vi "Test2.vi"(6 "Value":sgl=6.6666, 8 "Path":string=":NUMX", 9 "Mode":string="EDIT", 10 "Shot":i32=-1, 11 "Name":string="my_tree") -> (3 "Float out":sgl)   [LabVIEW 2010]
uses:
  <vilib>/MDSplus/Classes/Tree_Class/Tree.lvclass
  <vilib>/MDSplus/Classes/Data_Class/Scalar_Class/Float32_Class/Float32.lvclass
  <vilib>/MDSplus/Classes/Data_Class/Data.lvclass
  <vilib>/MDSplus/Classes/Data_Class/TreeNode_Class/TreeNode.lvclass
panel:
  out "error out":errorcluster
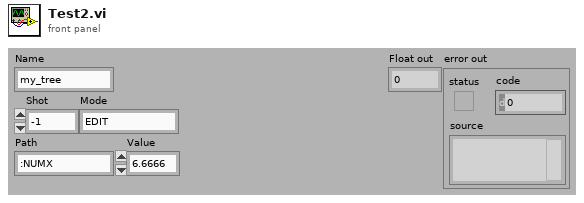
[diagram p1: front panel]
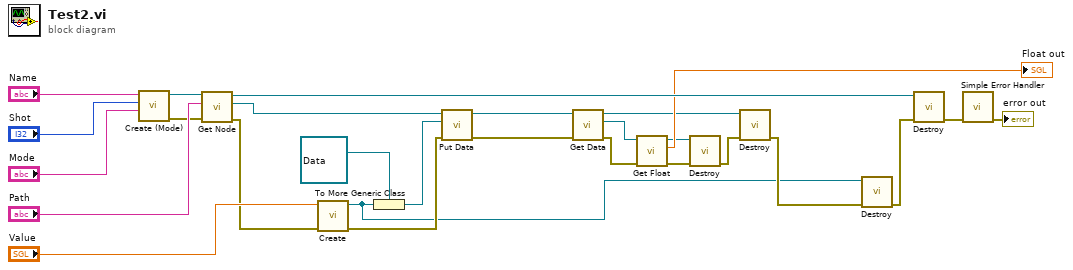
[diagram p0: block diagram]
diagram:
  n1 = call <vilib>:"Create (Mode).vi"("Mode"="Mode", "Shot"="Shot", "Name"="Name") -> ("error out"=w20:errorcluster, "Tree out"=w21:refnum<class "Tree.lvclass">)  [unwired: 7 in]
  n2 = call-dynamic "Get Node.vi"("error in (no error)"=w20, "Path"="Path", "Tree in"=w21) -> ("error out"=w13:errorcluster, "Node out"=w19:refnum<class "TreeNode.lvclass">, "Tree out"=w23:refnum<class "Tree.lvclass">)  [unwired: 6 in]
  n3 = call <vilib>:"Create.vi"("error in (no error)"=w13, "SGL in"="Value") -> ("error out"=w12:errorcluster, "Float32 out"=w1:refnum<class "Float32.lvclass">)  [unwired: 8 in]
  n4 = To More Generic Class(target class=refnum<class "Data.lvclass"> refnum ("Data.lvclass"), reference=w1) -> (generic class reference=w16:refnum<class "Data.lvclass">)
  n5 = call-dynamic "Put Data.vi"("error in (no error)"=w12, "Data"=w16, "TreeNode in"=w19) -> ("error out"=w5:errorcluster, "TreeNode out"=w15:refnum<class "TreeNode.lvclass">)  [unwired: 7 in]
  n6 = call-dynamic "Get Data.vi"("error in (no error)"=w5, "TreeNode in"=w15) -> ("error out"=w14:errorcluster, "Data out"=w2:refnum<class "Data.lvclass">, "TreeNode out"=w8:refnum<class "TreeNode.lvclass">)  [unwired: 7 in]
  n7 = call-dynamic "Get Float.vi"("error in (no error)"=w14, "Data in"=w2) -> ("error out"=w9:errorcluster, "SGL out"=→"Float out":sgl, "Data out"=w10:refnum<class "Data.lvclass">)  [unwired: 7 in]
  n8 = call-dynamic "Destroy.vi"("error in (no error)"=w9, "Data in"=w10) -> ("error out"=w7:errorcluster)  [unwired: 9 in]
  n9 = call-dynamic "Destroy.vi"("error in (no error)"=w7, "TreeNode in"=w8) -> ("error out"=w3:errorcluster)  [unwired: 9 in]
  n10 = call-dynamic "Destroy.vi"("error in (no error)"=w3, "Float32 in"=w1) -> ("error out"=w6:errorcluster)  [unwired: 9 in]
  n11 = call-dynamic "Destroy.vi"("error in (no error)"=w6, "Tree in"=w23) -> ("error out"=w22:errorcluster)  [unwired: 8 in]
  n12 = call <vilib>:"Simple Error Handler.vi"("error in (no error)"=w22) -> ("error out"=→"error out":errorcluster)  [unwired: 4 in, 4 out]
